vi "G Union to PLC Byte Stream.vi"(6 "Byte Length":i32, 8 "error in (no error)":errorcluster, 10 "Value":variant, 11 "TwinCAT ADS in":refnum<class "TwinCAT ADS.lvclass">) -> (0 "error out":errorcluster, 2 "Byte Stream":u8[](array[numeric]), 3 "TwinCAT ADS out":refnum<class "TwinCAT ADS.lvclass">)   [LabVIEW 2018, in "TwinCAT ADS.lvclass"]
uses:
  TwinCAT ADS.lvclass
  G Primitive to PLC Byte Stream.vi/ebfc1059-5ad7-41af-9a32-6ba056cec1e2.vi
  G Primitive to PLC Byte Stream.vi/6e01a951-886b-41b5-8cd1-fdd71fd1a533.vi
  G Primitive to PLC Byte Stream.vi/09c7a0ef-3209-4624-b801-f77696e71225.vi
  G Primitive to PLC Byte Stream.vi/97b8602c-6a72-408e-90bf-08a26de32539.vi
  G Primitive to PLC Byte Stream.vi/0fd4fbf3-4a18-432c-8f70-6a5c8fef8454.vi
  G Primitive to PLC Byte Stream.vi/afdb5a5e-237c-4be5-828e-15f510cf6cea.vi
  G Primitive to PLC Byte Stream.vi/185a6e12-4d7d-4ad7-9936-0525adb2f85e.vi
  G Primitive to PLC Byte Stream.vi/88229fb8-b58c-494b-bd2b-fea6e0d0ed1b.vi
  G Primitive to PLC Byte Stream.vi/e57df404-389c-41d0-a67c-37c75754ab31.vi
  G Primitive to PLC Byte Stream.vi/d0ee652c-9b86-46ed-9065-57d03aa8de3e.vi
  G Primitive to PLC Byte Stream.vi/886bf0b9-f01c-4a44-b2e2-abccc7b97bfa.vi
  G Primitive to PLC Byte Stream.vi/35f71df7-fc14-4c4d-983c-cf72c138dc9e.vi
  G Primitive to PLC Byte Stream.vi/2d2bc992-a9ff-4dd8-b8fe-74c21cb85899.vi
  G Primitive to PLC Byte Stream.vi/100e4a11-5e4a-45b7-be98-adc9eaebd48d.vi
  G Primitive to PLC Byte Stream.vi/132946d9-68c7-4ade-a66d-dc369520c644.vi
  <vilib>/Utility/error.llb/Error Cluster From Error Code.vi
  <vilib>/Utility/error.llb/Trim Whitespace.vi
  <vilib>/ErrorRing/Error Ring.xnode
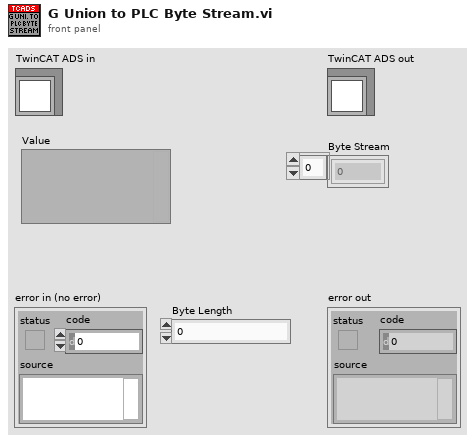
[diagram p1: front panel]
types:
  T1 = typedef "TwinCAT ADS.lvclass/PLC Type.ctl" = enum16{"UNDEFINED", "INT", "DINT", "REAL", "LREAL", "SINT", "BYTE", "UINT", "UDINT", "LINT", "ULINT", "STRING", "WSTRING", "BOOL", "TIME", "LTIME", "DATE", "DT", "TOD", "ARRAY", "JAGGED ARRAY", "STRUCT", "FUNCTION BLOCK", "UNION", "POINTER", "USER DEFINED"}
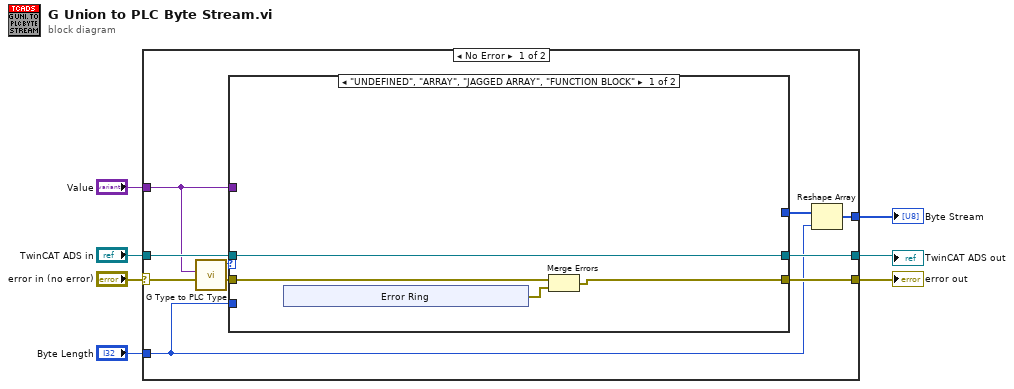
[diagram p0: block diagram]
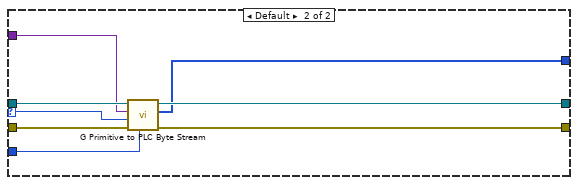
[diagram p2: hidden frame]
diagram:
  n1 = case shown="No Error" "error in (no error)" {
    selector: "error in (no error)" -> [w10 w35]
    tunnel: [w15 w35] -> w6
    tunnel: "Value" -> [w11 _]
    tunnel: "Byte Length" -> [w12 _]
    tunnel: [w17 _] -> w1
    tunnel: "TwinCAT ADS in" -> [w16 w34]
    tunnel: [w14 w34] -> w2
    frame No Error {
      n2 = call "G Type to PLC Type.vi"("error in (no error)"=w10, "Variant In"=w11) -> ("error out"=w9:errorcluster, "PLC Type"=w8:T1)  [unwired: 8 in]
      n3 = case shown="\"UNDEFINED\", \"ARRAY\", \"JAGGED ARRAY\", \"FUNCTION BLOCK\"" w8 {
        selector: w8 -> [_ w32]
        tunnel: w16 -> [w21 w33]
        tunnel: [w18 w31] -> w15
        tunnel: [w21 w30] -> w14
        tunnel: [_ w29] -> w13
        tunnel: w11 -> [_ w28]
        tunnel: w12 -> [_ w27]
        tunnel: w9 -> [w20 w26]
        frame "UNDEFINED", "ARRAY", "JAGGED ARRAY", "FUNCTION BLOCK" {
          n4 = xnode "Error Ring"() -> ("error out"=w19:errorcluster)
          n5 = Merge Errors(w20, w19) -> (w18:errorcluster)
        }
        frame Default {
          n6 = call "G Primitive to PLC Byte Stream.vi"("Byte Length"=w27, "error in (no error)"=w26, "PLC Type"=w32, "Value"=w28, "TwinCAT ADS in"=w33) -> ("error out"=w31:errorcluster, "Byte Stream"=w29:u8[], "TwinCAT ADS out"=w30:refnum<class "TwinCAT ADS.lvclass">)  [unwired: 4 in]
        }
      }
      n7 = Reshape Array(w13, w12) -> (w17:u8[])
    }
    frame Error {
    }
  }
  "error out" <- w6
  "TwinCAT ADS out" <- w2
  "Byte Stream" <- w1
